vi "SpecA_ESA_MatchIDNStr.vi"(8 "error in (no error)":errorcluster, 10 "IDNStr":string) -> (0 "error out":errorcluster, 2 "IDN match":bool, 3 "ClassLibraryFile":path)   [LabVIEW 2014]
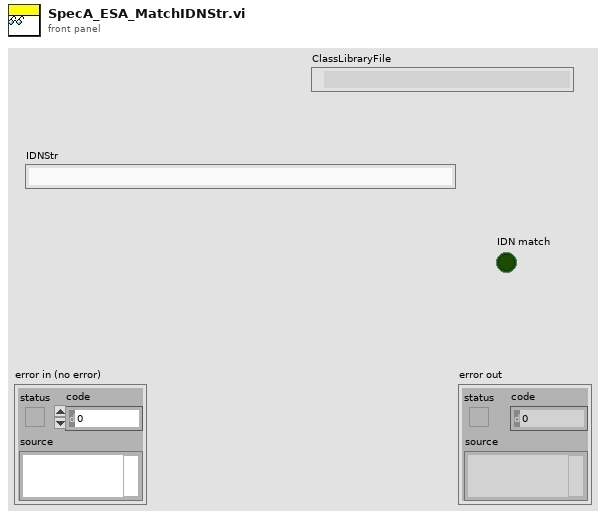
[diagram p1: front panel]
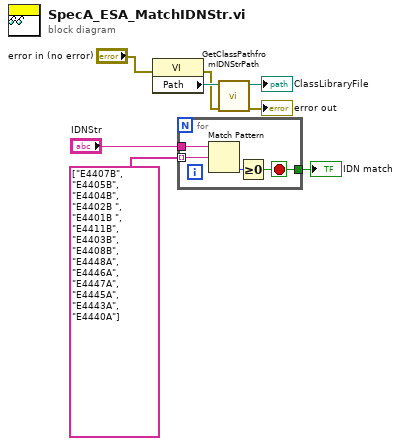
[diagram p0: block diagram]
diagram:
  n1 = property class="VI"(error in="error in (no error)") -> (error out=w4:errorcluster, "Path"=w7:path)  [unwired: 1 in, 1 out]
  n2 = for {
    tunnel: [w12] -> w3
    tunnel: "IDNStr" -> [w11]
    tunnel: string[] ["E4407B", "E4405B", "E4404B", "E4402B ", "E4401B ", "E4411B", "E4403B", "E4408B", "E4448A", "E4446A", "E4447A", "E4445A", "E4443A", "E4440A"] -> [w9] mode=indexing
    stop <- w12 stop-if-true
    n3 = Match Pattern(string=w11, regular expression=w9) -> (offset past match=w10:i32)  [unwired: 1 in, 3 out]
    n4 = Greater Or Equal To 0?(x=w10) -> (x >= 0?=w12:bool)
  }
  "IDN match" <- w3
  n5 = call "GetClassPathfromIDNStrPath.vi"("error in (no error)"=w4, "Path in"=w7) -> ("error out"=→"error out":errorcluster, "Path out"=→"ClassLibraryFile":path)  [unwired: 8 in]
